vi "Set Offset Tuning state.vi"(8 "error in (no error)":errorcluster, 10 "Offset Tuning":bool, 11 "DeviceRefnum":u64) -> (0 "error out":errorcluster, 2 "function return":i32, 3 "DeviceRefnum Out":u64)   [LabVIEW 2016]
doc: "Enable or disable offset tuning for zero-IF tuners, which allows to avoid problems caused by the DC offset of the ADCs and 1/f noise."
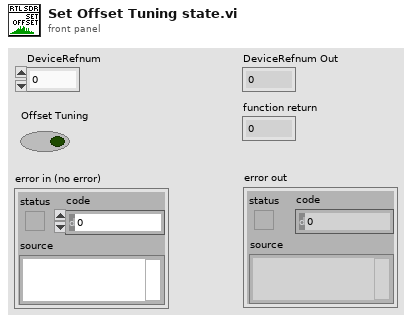
[diagram p1: front panel]
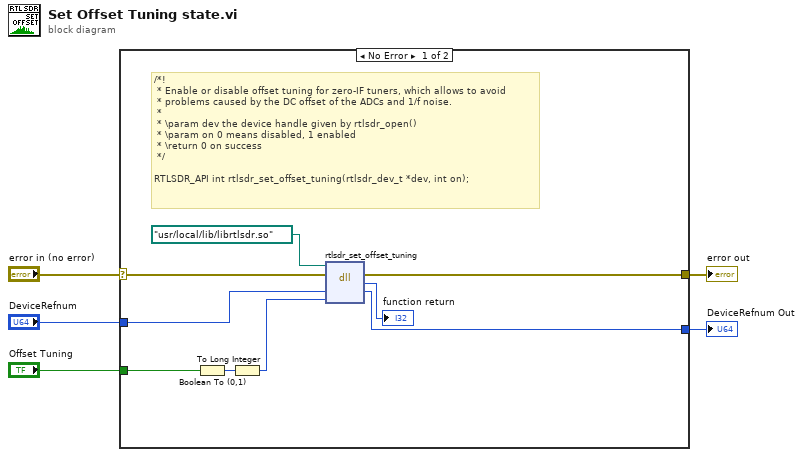
[diagram p0: block diagram]
diagram:
  n1 = case shown="No Error" "error in (no error)" {
    selector: "error in (no error)" -> [w7 w16]
    tunnel: [w13 w16] -> w5
    tunnel: "DeviceRefnum" -> [w12 w15]
    tunnel: [w11 w15] -> w3
    tunnel: "Offset Tuning" -> [w9 _]
    frame No Error {
      # "/*!\n * Enable or disable offset tuning for zero-IF tuners, which allows to avoid\n * problems caused by the DC offset of the ADCs and 1/f noise.\n *\n * \\param dev the device handle given by rtlsdr_open()\n * \\param on 0 means disabled, 1 enabled\n * \\return 0 on success\n */\n\nRTLSDR_API int rtlsdr_set_offset_tuning(rtlsdr_dev_t *dev, int on);"
      n2 = Boolean To (0,1)(Boolean=w9) -> (0, 1=w10:i16)
      n3 = To Long Integer(number=w10) -> (32bit integer=w8:i32)
      n4 = dll-call lib="C:/Program Files (x86)/National Instruments/LabVIEW 2016/user.lib/rtlsdr/rtlsdr.*" fn="rtlsdr_set_offset_tuning"(path in=path "/usr/local/lib/librtlsdr.so", error in=w7, "DeviceRefnum"=w12, "Offset Tuning"=w8) -> (error out=w13:errorcluster, "return type"=→"function return":i32, "DeviceRefnum"=w11:u64)  [unwired: 2 in, 1 out]
    }
    frame Error {
    }
  }
  "error out" <- w5
  "DeviceRefnum Out" <- w3
